vi "ROI.vi"(0 "image in":refnum<class "MSC Image.lvclass">, 1 "ROIs In":T1[](array[typedef]) {"Type" items=["Point", "Line", "Rectangle", "Oval", "Freehand / Polygon"]}, 2 "ROI ID":dbl=nan format="%#_13g", 5 "error in (no error)":errorcluster, 8 "Crop?":bool) -> (14 "image out":refnum<class "MSC Image.lvclass">, 15 "ROIs Out":T1[](array[typedef]) {"Type" items=["Point", "Line", "Rectangle", "Oval", "Freehand / Polygon"]}, 16 "particle image out":refnum<class "MSC Image.lvclass">, 17 "particle mask image out":refnum<class "MSC Image.lvclass">, 19 "error out":errorcluster)   [LabVIEW 2014, in "MSC Image.lvclass"]
doc: "Calculates the Region Of Interest of the image. \nIf there is hierarchy information present (e.g. from \"Calculate Contours\"), the ROI doesnt contain its children.\nWire the ROI ID from \"ROI - Fill Tree\" to display only the selected ROI. \nCrop crops the ROI image to its bounding box.\n\"IMAQ ROI to MSC Image ROI\" is useful when you want to use a IMAQ Control to select the ROIs."
uses:
  MSC Image.lvclass
  controls/ROI.ctl
  controls/ROI Type.ctl
  controls/Contour.ctl
  controls/Contour hierarchy.ctl
  controls/Size.ctl
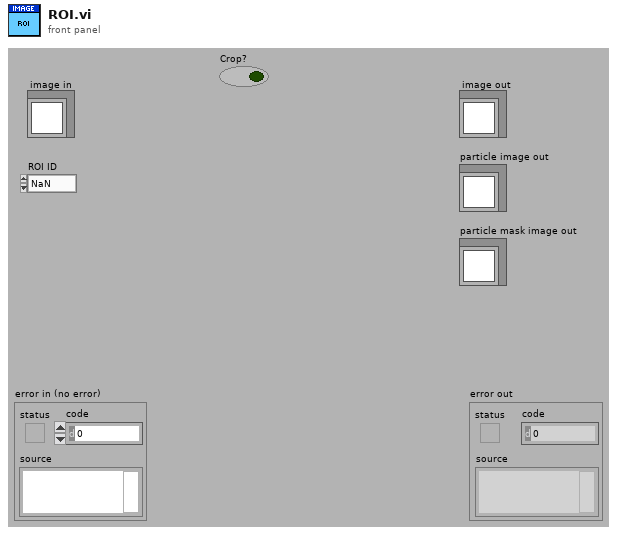
[diagram p1: front panel]
types:
  T1 = typedef "MSC Image.lvclass/ROI.ctl" = cluster{"Type":T2, "Parameters":dbl[], "Contour":T3, "Bounding Box":T3, "Contour Length":dbl, "ROI Area":dbl, "ROI Mean":dbl, "ROI Standard Deviation":dbl, "ROI Min":dbl, "ROI Max":dbl, "Hierarchy":T4, "Variant":variant, "Timestamp":timestamp}
  T2 = typedef "MSC Image.lvclass/ROI Type.ctl" = u16
  T3 = typedef "MSC Image.lvclass/Contour.ctl" = cluster{"x":i16, "y":i16}[]
  T4 = typedef "MSC Image.lvclass/Contour hierarchy.ctl" = cluster{"parent ID":i32, "children IDs":dbl[], "level":i32}
  T5 = typedef "MSC Image.lvclass/Size.ctl" = cluster{"Cols":i32, "Rows":i32}
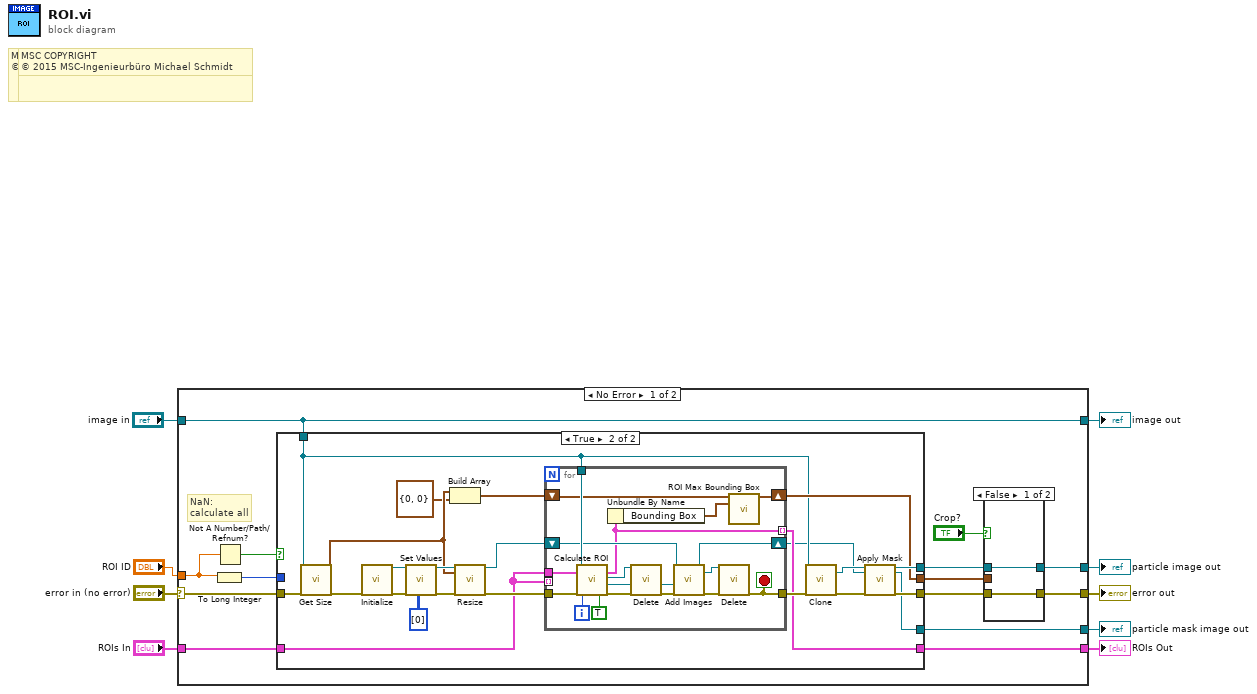
[diagram p0: block diagram]
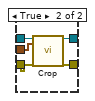
[diagram p2: hidden frame]
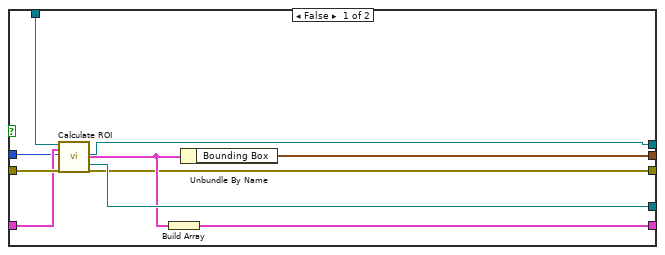
[diagram p3: hidden frame]
diagram:
  # "MSC COPYRIGHT\n© 2016 MSC-Ingenieurbüro Michael Schmidt"
  # "MSC COPYRIGHT\n© 2016 MSC-Ingenieurbüro Michael Schmidt"
  # "MSC COPYRIGHT\n© 2015 MSC-Ingenieurbüro Michael Schmidt"
  # "MSC COPYRIGHT\n© 2015 MSC-Ingenieurbüro Michael Schmidt"
  n1 = case shown="No Error" "error in (no error)" {
    selector: "error in (no error)" -> [w23 w83]
    tunnel: [w16 w84] -> w7
    tunnel: "image in" -> [w16 w84]
    tunnel: [w21 w83] -> w6
    tunnel: [w18 _] -> w3
    tunnel: "ROIs In" -> [w17 w82]
    tunnel: [w14 _] -> w4
    tunnel: [w13 w82] -> w2
    tunnel: "ROI ID" -> [w12 _]
    frame No Error {
      # "NaN:\ncalculate all"
      n2 = To Long Integer(number=w12) -> (32bit integer=w10:i32)
      n3 = Not A Number/Path/Refnum?(number/path/refnum=w12) -> (NaN/Path/Refnum?=w11:bool)
      n4 = case shown="True" w11 {
        tunnel: [w33 w53] -> w22
        tunnel: w23 -> [w40 w54]
        tunnel: w16 -> [w37 w43]
        tunnel: [w39 w46] -> w20
        tunnel: [w38 w47] -> w19
        tunnel: [w36 w45] -> w18
        tunnel: [w34 w44] -> w13
        tunnel: w17 -> [w32 w48]
        tunnel: w10 -> [w31 _]
        frame False {
          n5 = call "Calculate ROI.vi"("image in"=w37, "ROIs In"=w32, "ROI ID"=w31, "error in (no error)"=w40) -> ("ROI"=w35:T1, "particle image out"=w38:refnum<class "MSC Image.lvclass">, "particle mask image out"=w36:refnum<class "MSC Image.lvclass">, "error out"=w33:errorcluster)  [unwired: 11 in, 1 out]
          n6 = Build Array(w35) -> (w34:T1[])
          n7 = Unbundle By Name(w35) -> ("Bounding Box"=w39:T3)
        }
        frame True {
          n8 = call-dynamic "Get Size.vi"("image in"=w43, "error in (no error)"=w54) -> ("Size"=w52:T5, "error out"=w60:errorcluster)  [unwired: 15 in, 1 out]
          n9 = call "Initialize.vi"("error in (no error)"=w60) -> ("image out"=w55:refnum<class "MSC Image.lvclass">, "error out"=w59:errorcluster)  [unwired: 17 in]
          n10 = call-dynamic "Set Values.vi"("image in"=w55, "imageData U8"=u8[][] [[0]], "error in (no error)"=w59) -> ("image out"=w63:refnum<class "MSC Image.lvclass">, "error out"=w62:errorcluster)  [unwired: 15 in]
          n11 = Build Array(w52, T5 {"Cols"=0, "Rows"=0} ("Size")) -> (w51:T5[])
          n12 = call-dynamic "Resize.vi"("image in"=w63, "Size"=w52, "error in (no error)"=w62) -> ("image out"=w49:refnum<class "MSC Image.lvclass">, "error out"=w58:errorcluster)  [unwired: 15 in]
          n13 = for {
            tunnel: w43 -> [w77]
            shift-right: [w66] -> w46
            shift-left: w51 -> [w67]
            shift-right: [w64] -> w41
            shift-left: w49 -> [w72]
            tunnel: w48 -> [w76]
            tunnel: w48 -> [_] mode=indexing
            tunnel: w58 -> [w81]
            tunnel: [w69] -> w57
            tunnel: [w68] -> w44 mode=indexing
            i -> [w75]
            stop <- w69 stop-if-true
            n14 = call "Calculate ROI.vi"("image in"=w77, "ROIs In"=w76, "ROI ID"=w75, "error in (no error)"=w81, "Keep images?"=TRUE) -> ("ROI"=w68:T1, "particle image out"=w73:refnum<class "MSC Image.lvclass">, "particle mask image out"=w70:refnum<class "MSC Image.lvclass">, "error out"=w80:errorcluster)  [unwired: 10 in, 1 out]
            n15 = Unbundle By Name(w68) -> ("Bounding Box"=w65:T3)
            n16 = call-dynamic "Delete.vi"("image in"=w73, "error in (no error)"=w80) -> ("error out"=w79:errorcluster)  [unwired: 17 in]
            n17 = call-dynamic "Add Images.vi"("image in"=w72, "image 2 in"=w70, "error in (no error)"=w79) -> ("image out"=w64:refnum<class "MSC Image.lvclass">, "image 2 out"=w71:refnum<class "MSC Image.lvclass">, "error out"=w78:errorcluster)  [unwired: 14 in]
            n18 = call-dynamic "Delete.vi"("image in"=w71, "error in (no error)"=w78) -> ("error out"=w69:errorcluster)  [unwired: 17 in]
            n19 = call "ROI Max Bounding Box.vi"("Bounding Box In 1"=w67, "Bounding Box In 2"=w65) -> ("Max Bounding Box"=w66:T3)  [unwired: 13 in]
          }
          n20 = call-dynamic "Clone.vi"("image in"=w43, "error in (no error)"=w57) -> ("clone image out"=w42:refnum<class "MSC Image.lvclass">, "error out"=w56:errorcluster)  [unwired: 15 in, 1 out]
          n21 = call-dynamic "Apply Mask.vi"("image in"=w42, "mask image in"=w41, "error in (no error)"=w56) -> ("image out"=w47:refnum<class "MSC Image.lvclass">, "mask image out"=w45:refnum<class "MSC Image.lvclass">, "error out"=w53:errorcluster)  [unwired: 14 in]
        }
      }
      n22 = case shown="False" "Crop?" {
        tunnel: w22 -> [w25 w30]
        tunnel: [w25 w29] -> w21
        tunnel: w20 -> [_ w28]
        tunnel: w19 -> [w24 w27]
        tunnel: [w24 w26] -> w14
        frame False {
        }
        frame True {
          n23 = call-dynamic "Crop.vi"("image in"=w27, "Bounding Box"=w28, "error in (no error)"=w30) -> ("image out"=w26:refnum<class "MSC Image.lvclass">, "error out"=w29:errorcluster)  [unwired: 14 in, 1 out]
        }
      }
    }
    frame Error {
    }
  }
  "error out" <- w6
  "image out" <- w7
  "particle image out" <- w4
  "particle mask image out" <- w3
  "ROIs Out" <- w2
